vi "BenchmarkSorting.vi"() -> ()   [LabVIEW 2014]
panel:
  out "input":dbl[](array[numeric])
  out "time_selection":u32
  out "time_insertion":u32
  out "time_bubble":u32
  out "selection sorted":dbl[](array[numeric])
  out "insertion sorted":dbl[](array[numeric])
  out "bubble sorted":dbl[](array[numeric])
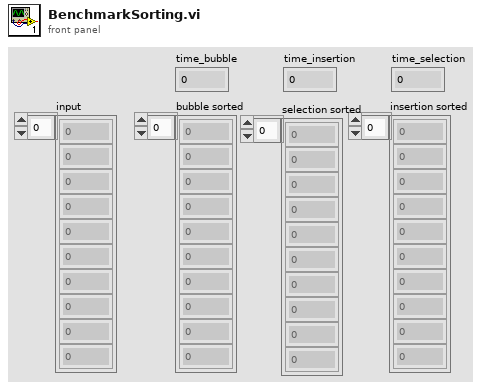
[diagram p1: front panel]
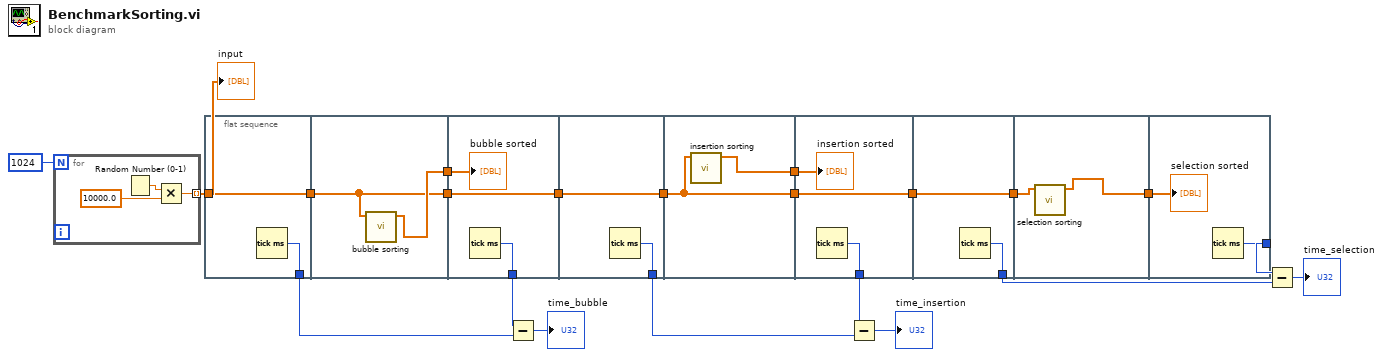
[diagram p0: block diagram]
diagram:
  n1 = for {
    N: 1024 -> [_]
    tunnel: [w22] -> w20 mode=indexing
    n2 = Random Number (0-1)() -> (number: 0 to 1=w24:dbl)
    n3 = Multiply(x=w24, y=10000.0) -> (x*y=w22:dbl)
  }
  "input" <- w20
  n4 = flat-sequence {
    tunnel: [w26] -> w16
    tunnel: w20 -> [w26]
    tunnel: [w25] -> w9
    tunnel: [w28] -> w19
    tunnel: [w27] -> w17
    tunnel: w16 -> [w27]
    tunnel: w19 -> [w31]
    tunnel: [w30] -> w15
    tunnel: w17 -> [w30]
    tunnel: [w29] -> w8
    tunnel: w15 -> [w33]
    tunnel: [w33] -> w14
    tunnel: [w32] -> w6
    tunnel: [w34] -> w18
    tunnel: w14 -> [w34]
    tunnel: [w35] -> w13
    tunnel: w18 -> [w38]
    tunnel: w13 -> [w37]
    tunnel: [w38] -> w12
    tunnel: [w36] -> w7
    tunnel: w12 -> [w40]
    tunnel: [w40] -> w11
    tunnel: [w39] -> w4
    tunnel: w11 -> [w41]
    tunnel: [w42] -> w10
    tunnel: w10 -> [w44]
    tunnel: [w43] -> w5
    frame #0 {
      n5 = Tick Count (ms)() -> (millisecond timer value=w25:u32)
    }
    frame #1 {
      n6 = call "bubble sorting.vi"("Array"=w27) -> ("sorted"=w28:dbl[])  [unwired: 9 in]
    }
    frame #2 {
      n7 = Tick Count (ms)() -> (millisecond timer value=w29:u32)
      "bubble sorted" <- w31
    }
    frame #3 {
      n8 = Tick Count (ms)() -> (millisecond timer value=w32:u32)
    }
    frame #4 {
      n9 = call "insertion sorting.vi"("input"=w34) -> ("sorted"=w35:dbl[])  [unwired: 10 in]
    }
    frame #5 {
      n10 = Tick Count (ms)() -> (millisecond timer value=w36:u32)
      "insertion sorted" <- w37
    }
    frame #6 {
      n11 = Tick Count (ms)() -> (millisecond timer value=w39:u32)
    }
    frame #7 {
      n12 = call "selection sorting.vi"("input"=w41) -> ("sorted"=w42:dbl[])  [unwired: 10 in]
    }
    frame #8 {
      n13 = Tick Count (ms)() -> (millisecond timer value=w43:u32)
      "selection sorted" <- w44
    }
  }
  n14 = Subtract(x=w8, y=w9) -> (x-y=→"time_bubble":u32)
  n15 = Subtract(x=w7, y=w6) -> (x-y=→"time_insertion":u32)
  n16 = Subtract(x=w5, y=w4) -> (x-y=→"time_selection":u32)
